vi "CRLF.vi"() -> (0 "CRLF":string)   [LabVIEW 2015, in "MJPEG Reader.lvclass"]
uses:
  MJPEG Reader.lvclass
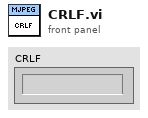
[diagram p1: front panel]
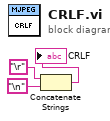
[diagram p0: block diagram]
diagram:
  n1 = Concatenate Strings("\r", "\n") -> (→"CRLF":string)
